vi "ConnectionInfoUpdated.vi"(8 "error in (no error)":errorcluster, 10 "Connection Information":T1={"Connection number"=-1, "Remote Address"="", "Remote Port"=0, "Connection ID"=refnum, "bytes received"=0, "bytes  sent"=0}, 11 "TCP_Server in":refnum<class "TCP_Server.lvclass">) -> (0 "error out":errorcluster, 3 "TCP_Server out":refnum<class "TCP_Server.lvclass">)   [LabVIEW 2023, in "TCP_Server.lvlib" / "TCP_Server.lvclass"]
uses:
  TCP_Server.lvclass
  TCP_Server.lvclass/TCP_Server.ctl
  TCP_Server Messages/UpdateGUIconnectionTable Msg/UpdateGUIconnectionTable Msg.lvclass
  <vilib>/ActorFramework/Actor/Actor.lvclass
  C:/Program Files (x86)/National Instruments/LabVIEW 2023/vi.lib/ActorFramework/Actor/Actor.lvclass
  C:/Source/LabVIEW/TCP_server/TCP_Server/TCP_Server/TCP_Server.lvclass
  C:/Source/LabVIEW/TCP_server/SimpleErrorLogger/ApplicationWithErrorLogger/ApplicationWithErrorLogger.lvclass
  C:/Source/LabVIEW/TCP_server/TCP_Client_Window/TCP_ClientWindow_Controller/TCP_ClientWindow_Controller.lvclass
  C:/Source/LabVIEW/TCP_server/TCP_Listener/Connections Controller/Connections Controller.lvclass
  C:/Source/LabVIEW/TCP_server/TCP_Server_Connection_Handler/TCP_Connections_Controller/TCP_Connections_Controller.lvclass
  C:/Source/LabVIEW/TCP_server/TCP_serverGUI/TCP_ServerWithGUI/TCP_ServerWithGUI.lvclass
  TCP_Listener/TypeDefinitions/ConnectionInformation.ctl
  TCP_Listener/TCP_Listener.lvlib
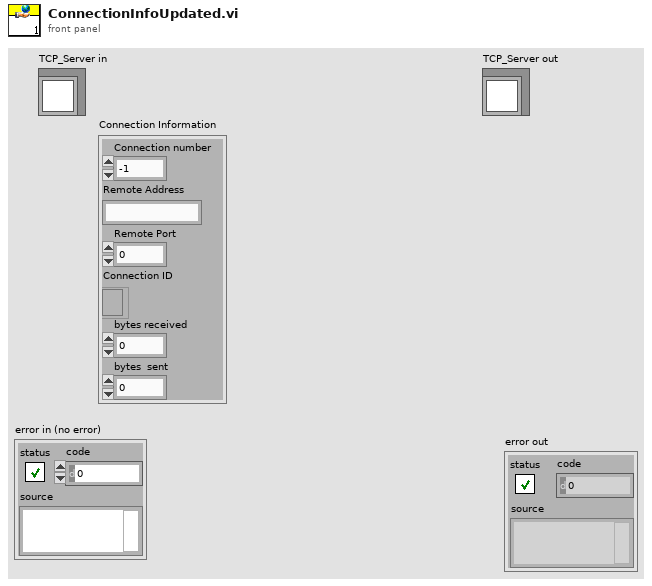
[diagram p1: front panel]
types:
  T1 = typedef "TCP_Listener.lvlib/ConnectionInformation.ctl" = cluster{"Connection number":i32, "Remote Address":string, "Remote Port":u16, "Connection ID":refnum<k5>, "bytes received":i32, "bytes  sent":i32}
  T2 = typedef "TCP_Server.lvlib/ServerConnection.ctl" = cluster{"Connection Handlers's Enqueuer":refnum<class "Message Enqueuer.lvclass">, "Connection Window's Enqueuer":refnum<class "Message Enqueuer.lvclass">, "Connection Information":T1}
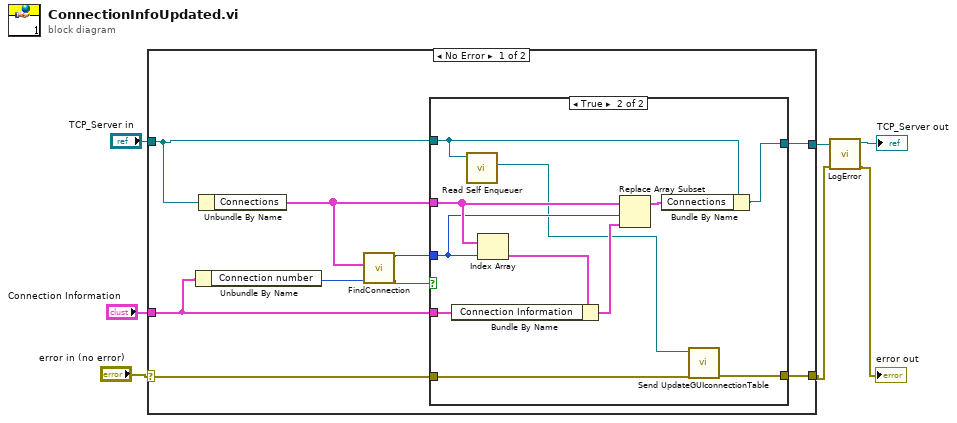
[diagram p0: block diagram]
diagram:
  n1 = case shown="No Error" "error in (no error)" {
    selector: "error in (no error)" -> [w9 w31]
    tunnel: [w8 w31] -> w2
    tunnel: "TCP_Server in" -> [w11 w30]
    tunnel: [w10 w30] -> w4
    tunnel: "Connection Information" -> [w12 _]
    frame No Error {
      n2 = Unbundle By Name(w12) -> ("Connection number"=w16:i32)
      n3 = Unbundle By Name(w11) -> ("Connections"=w13:T2[])
      n4 = call "FindConnection.vi"("Connection number"=w16, "Connections"=w13) -> ("Found?"=w15:bool, "Connection index"=w14:i32)  [unwired: 6 in, 2 out]
      n5 = case shown="True" w15 {
        tunnel: w14 -> [_ w28]
        tunnel: w13 -> [_ w29]
        tunnel: w12 -> [_ w26]
        tunnel: w11 -> [w18 w20]
        tunnel: [w18 w23] -> w10
        tunnel: w9 -> [w17 w22]
        tunnel: [w17 w21] -> w8
        frame False {
        }
        frame True {
          n6 = call <vilib>:"Read Self Enqueuer.vi"("Actor"=w20) -> ("Self Enqueuer"=w19:refnum<class "Message Enqueuer.lvclass">)  [unwired: 10 in]
          n7 = Index Array(array=w29, index=w28) -> (element=w27:T2)
          n8 = Bundle By Name(cluster=w27, "Connection Information"=w26) -> (w25:T2)
          n9 = Replace Array Subset(array=w29, new element=w25, index=w28) -> (w24:T2[])
          n10 = Bundle By Name(cluster=w20, "Connections"=w24) -> (w23:refnum<class "TCP_Server.lvclass">)
          n11 = call "Send UpdateGUIconnectionTable.vi"("error in (no error)"=w22, "Message Enqueuer"=w19) -> ("error out"=w21:errorcluster)  [unwired: 8 in, 1 out]
        }
      }
    }
    frame Error {
    }
  }
  n12 = call "LogError.vi"("error in (no error)"=w2, "TCP_Server in"=w4) -> ("error out"=→"error out":errorcluster, "TCP_Server out"=→"TCP_Server out":refnum<class "TCP_Server.lvclass">)  [unwired: 8 in]
